vi "SV Update Signal.vi"(0 "current configuration":refnum<class "SV Signal.lvclass">, 5 "new configuration":refnum<class "SV Signal.lvclass">, 11 "error in (no error)":errorcluster) -> (4 "updated configuration":refnum<class "SV Signal.lvclass">, 15 "error out":errorcluster)   [LabVIEW 2017, in "SV Signal.lvclass"]
doc: "Dynamically updates a signal that is being generated with the Signal Generation API. Wire the current signal configuration to <B>current configuration</B> and the new signal configuration to <B>new configuration</B>. Pass the <B>updated configuration</B> output to SV Signal (waveform) VI to initiate the update. Use this VI when you want to transition from one configuration to another without having to stop the generation."
uses:
  <vilib>/addons/_NISVFA/_Generation/Signal Generation/SV Signal/SV Signal.lvclass
  <vilib>/addons/_NISVFA/_Generation/Signal Generation/SV Signal/SV Signal.lvclass/SV Signal.ctl
  <vilib>/addons/_NISVFA/_Generation/Signal Generation/SV Signal/sv_Signal State Attribute.ctl
  <vilib>/addons/_NISVFA/_Generation/Signal Generation/SV Signal/sv_System Timing Model.ctl
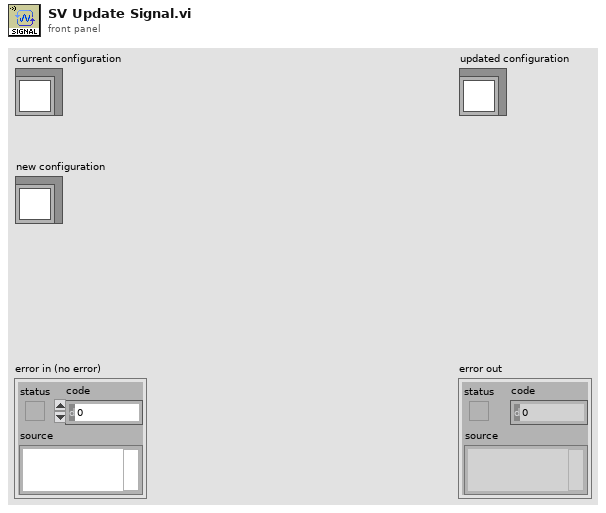
[diagram p1: front panel]
types:
  T1 = typedef "SV Signal.lvclass/sv_System Timing Model.ctl" = i64
  T2 = typedef "SV Signal.lvclass/sv_Generation State.ctl" = enum16{"Idle", "Ramp Up", "Pre-Measurement Settling", "Measurement", "Post-Measurement Settling", "Discrete Sweep Transition", "Ramp Down", "Update"}
  T3 = typedef "SV Signal.lvclass/sv_Signal State Attribute.ctl" = string
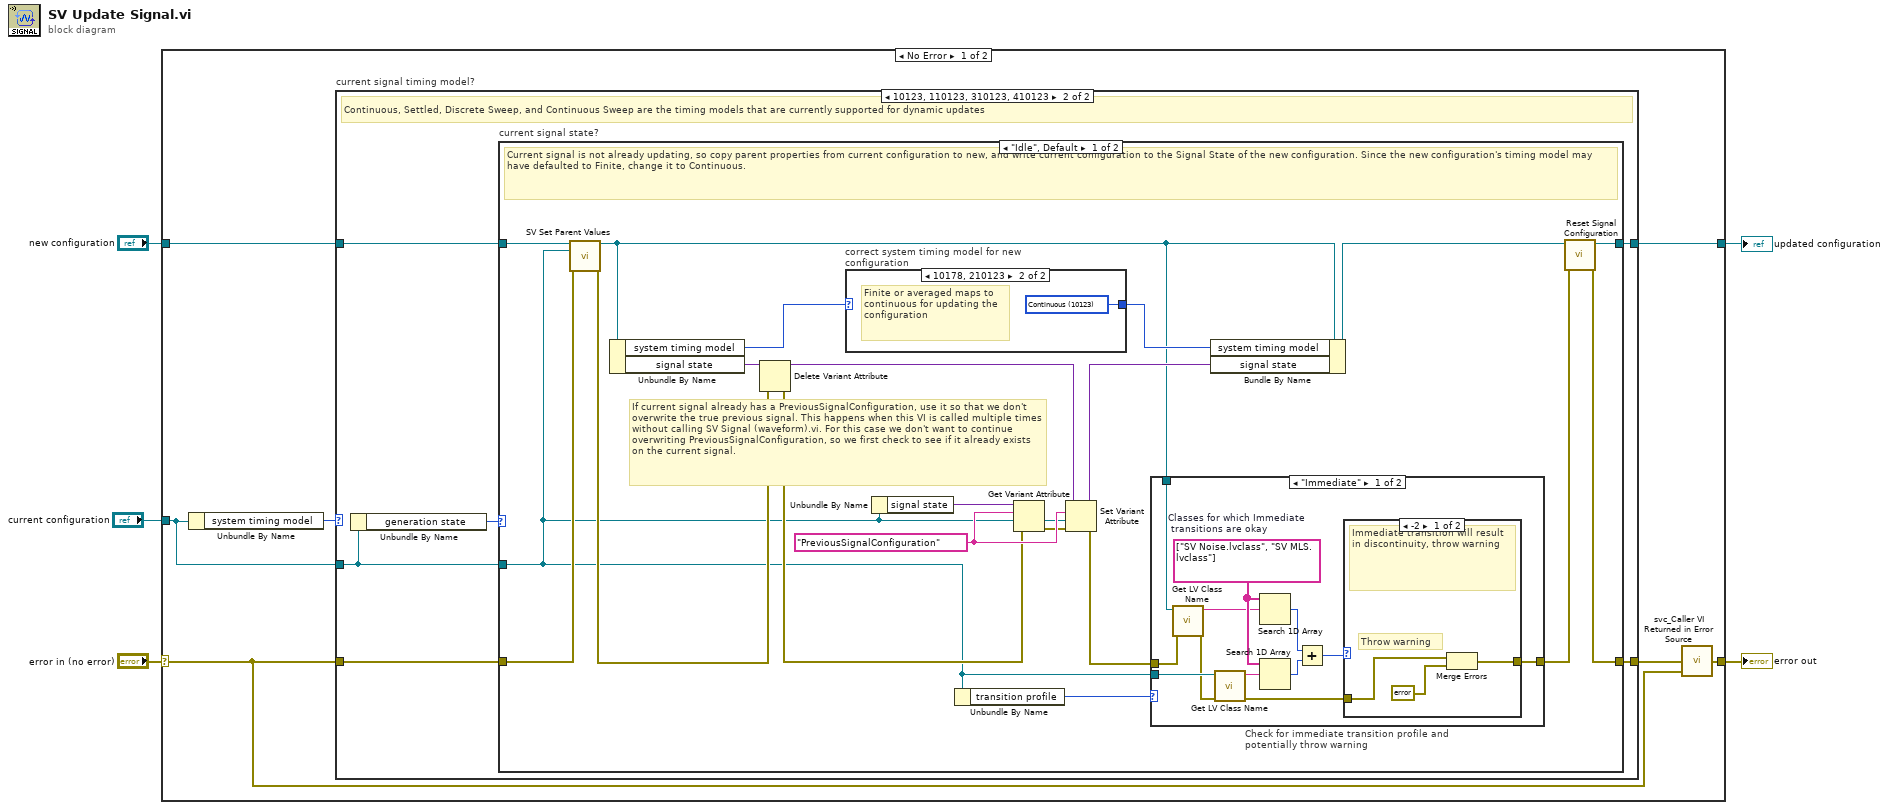
[diagram p0: block diagram]
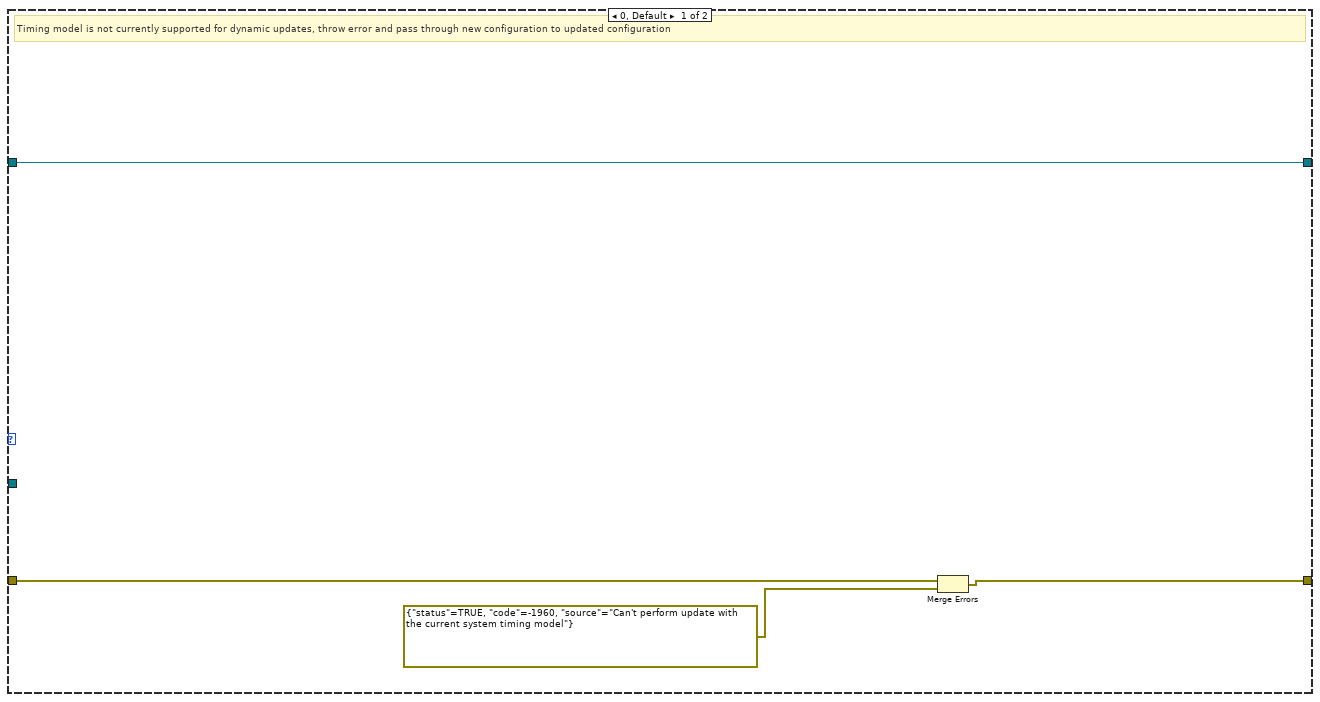
[diagram p2: hidden frame]
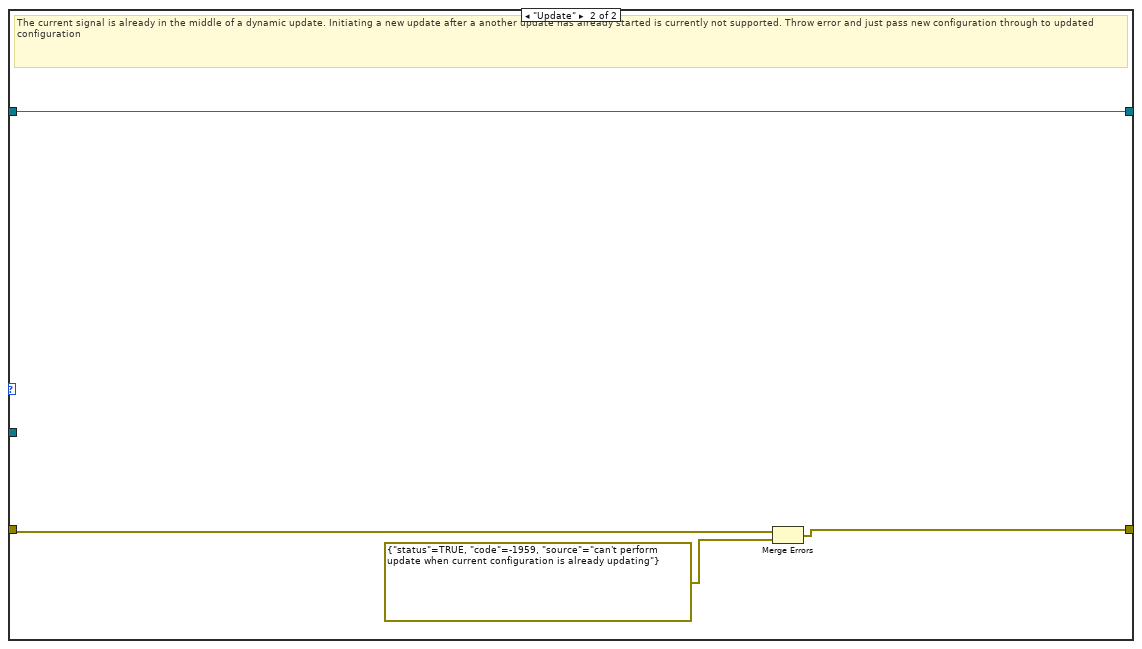
[diagram p6: hidden frame]
diagram:
  n1 = case shown="No Error" "error in (no error)" {
    selector: "error in (no error)" -> [w9 w67]
    tunnel: "new configuration" -> [w6 w68]
    tunnel: "current configuration" -> [w11 _]
    tunnel: [w7 w68] -> w3
    tunnel: [w10 w67] -> w2
    frame No Error {
      n2 = Unbundle By Name(w11) -> ("system timing model"=w12:T1)
      n3 = case "current signal timing model?" shown="10123, 110123, 310123, 410123" w12 {
        tunnel: w9 -> [w15 w22]
        tunnel: [w14 w21] -> w8
        tunnel: w11 -> [_ w19]
        tunnel: [w13 w18] -> w7
        tunnel: w6 -> [w13 w17]
        frame 0, Default {
          # "Timing model is not currently supported for dynamic updates, throw error and pass through new configuration to updated configuration"
          n4 = Merge Errors(w15, errorcluster {"status"=TRUE, "code"=-1960, "source"="Can't perform update with the current system timing model"} ("error out")) -> (w14:errorcluster)
        }
        frame 10123, 110123, 310123, 410123 {
          # "Continuous, Settled, Discrete Sweep, and Continuous Sweep are the timing models that are currently supported for dynamic updates"
          n5 = Unbundle By Name(w19) -> ("generation state"=w20:T2)
          n6 = case "current signal state?" shown="\"Idle\", Default" w20 {
            tunnel: w22 -> [w31 w66]
            tunnel: [w24 w64] -> w21
            tunnel: w19 -> [w28 _]
            tunnel: [w25 w63] -> w18
            tunnel: w17 -> [w32 w63]
            frame "Idle", Default {
              w42 = T3 "PreviousSignalConfiguration" ("name")
              # "If current signal already has a PreviousSignalConfiguration, use it so that we don't overwrite the true previous signal. This happens when this VI is called multiple times without calling SV Signal (waveform).vi. For this case we don't want to continue overwriting PreviousSignalConfiguration, so we first check to see if it already exists on the current signal."
              # "Current signal is not already updating, so copy parent properties from current configuration to new, and write current configuration to the Signal State of the new configuration. Since the new configuration's timing model may have defaulted to Finite, change it to Continuous."
              n7 = call-dynamic "SV Set Parent Values.vi"("child class in"=w32, "parent class"=w28, "error in (no error)"=w31) -> ("child class out"=w27:refnum<class "SV Signal.lvclass">, "error out"=w33:errorcluster)  [unwired: 11 in]
              n8 = Unbundle By Name(w27) -> ("system timing model"=w39:T1, "signal state"=w40:variant)
              n9 = Delete Variant Attribute(4:w33, 7:w40) -> (0:w35:errorcluster, 3:w37:variant)  [unwired: 1 in, 1 out]
              n10 = case "correct system timing model for new configuration" shown="10178, 210123" w39 {
                selector: w39 -> [w44 _]
                tunnel: [w44 w45] -> w38
                frame 0, Default {
                }
                frame 10178, 210123 {
                  w45 = T1 10123 items=["Finite"=10178, "-"=-1, "Continuous"=10123, "-"=-2, "Settled"=110123, "Averaged"=210123, "Discrete Sweep"=310123, "Continuous Sweep"=410123] ("system timing model")
                  # "Finite or averaged maps to continuous for updating the configuration"
                }
              }
              n11 = Unbundle By Name(w28) -> ("signal state"=w29:variant)
              n12 = Unbundle By Name(w28) -> ("transition profile"=w43:enum16{"Immediate", "Next optimum", "Ramp"})
              n13 = Get Variant Attribute(Variant=w29, name=w42, default value (empty Variant)=w28, error in=w35) -> (value=w36:refnum<class "SV Signal.lvclass">, error out=w34:errorcluster)  [unwired: 2 out]
              n14 = Set Variant Attribute(Variant=w37, name=w42, value=w36, error in=w34) -> (Variant out=w41:variant, error out=w30:errorcluster)  [unwired: 1 out]
              n15 = case "Check for immediate transition profile and potentially throw warning" shown="\"Immediate\"" w43 {
                tunnel: [w57 w62] -> w23
                tunnel: w30 -> [w50 w62]
                tunnel: w28 -> [w51 _]
                tunnel: w27 -> [w46 _]
                frame "Immediate" {
                  w54 = string[] ["SV Noise.lvclass", "SV MLS.lvclass"]  # Classes for which Immediate  transitions are okay
                  n16 = call <vilib>:"Get LV Class Name.vi"("error in (no error)"=w50, "object"=w46) -> ("error out"=w48:errorcluster, "class name"=w52:string)  [unwired: 8 in]
                  n17 = call <vilib>:"Get LV Class Name.vi"("error in (no error)"=w48, "object"=w51) -> ("error out"=w47:errorcluster, "class name"=w53:string)  [unwired: 8 in]
                  n18 = Search 1D Array(1D array=w54, element=w52) -> (index of element=w55:i32)  [unwired: 1 in]
                  n19 = Search 1D Array(1D array=w54, element=w53) -> (index of element=w56:i32)  [unwired: 1 in]
                  n20 = Add(x=w55, y=w56) -> (x+y=w49:i32)
                  n21 = case shown="-2" w49 {
                    tunnel: [w60 w61] -> w57
                    tunnel: w47 -> [w58 w61]
                    frame -2 {
                      # "Throw warning"
                      # "Immediate transition will result in discontinuity, throw warning"
                      n22 = Merge Errors(w58, errorcluster {"status"=FALSE, "code"=1959, "source"="possible discontinuity"} ("error in")) -> (w60:errorcluster)
                    }
                    frame 0, Default {
                      # "Don't throw warning if we are okay with immediate transition"
                    }
                  }
                }
                frame "Next optimum", "Ramp", Default {
                }
              }
              n23 = Bundle By Name(cluster=w27, "system timing model"=w38, "signal state"=w41) -> (w26:refnum<class "SV Signal.lvclass">)
              n24 = call-dynamic "Reset Signal Configuration.vi"("error in (no error)"=w23, "signal configuration in"=w26) -> ("error out"=w24:errorcluster, "signal configuration out"=w25:refnum<class "SV Signal.lvclass">)  [unwired: 8 in]
            }
            frame "Update" {
              # "The current signal is already in the middle of a dynamic update. Initiating a new update after a another update has already started is currently not supported. Throw error and just pass new configuration through to updated configuration"
              n25 = Merge Errors(w66, errorcluster {"status"=TRUE, "code"=-1959, "source"="can't perform update when current configuration is already updating"} ("error out")) -> (w64:errorcluster)
            }
          }
        }
      }
      n26 = call <vilib>:"svc_Caller VI Returned in Error Source.vi"("warning input to caller"=w9, "error in (no error)"=w8) -> ("error out"=w10:errorcluster)  [unwired: 3 in]
    }
    frame Error {
    }
  }
  "error out" <- w2
  "updated configuration" <- w3
